vi "Initialize File Transfer Behavior.vi"(8 "error in (no error)":errorcluster, 11 "RT Management in":refnum<class "RT Management.lvclass">) -> (0 "error out":errorcluster, 2 "File Transfer Behavior out":refnum<class "File Transfer Behavior.lvclass">, 3 "RT Management out":refnum<class "RT Management.lvclass">)   [LabVIEW 2016, in "RT Management.lvlib" / "RT Management.lvclass"]
doc: "Initializes the appropriate File Transfer Behavior for the given target."
uses:
  RT Management.lvclass
  File Transfer Behavior/File Transfer Behavior.lvclass
  RT Management.lvclass/RT Management.ctl
  FTP/FTP.lvclass
  C:/GitHub/SystemManagementAndInformation/source/classes/File Transfer Behavior/File Transfer Behavior.lvclass
  WebDAV/WebDAV.lvclass
  Get File transfer behavior.vi
  Get Password.vi
  Get Username.vi
  Get Address.vi
  Set File Transfer Behavior.lvclass.vi
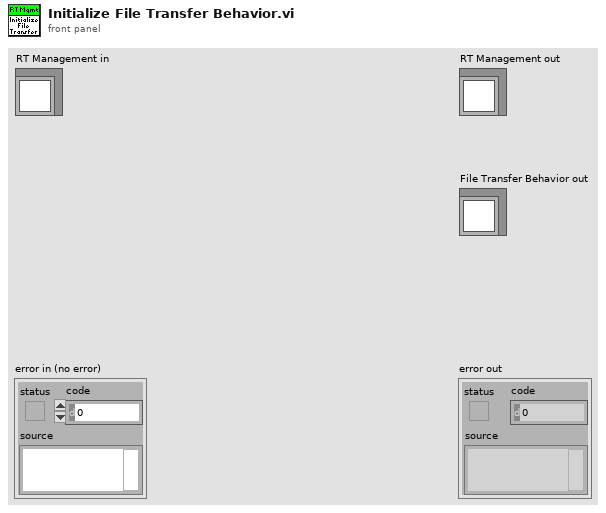
[diagram p1: front panel]
types:
  T1 = typedef "RT Management.lvlib/RT Management.lvclass/Operating system.ctl" = enum16{"Unknown", "VxWorks", "PharLap", "Linux-ARM", "Linux-x64"}
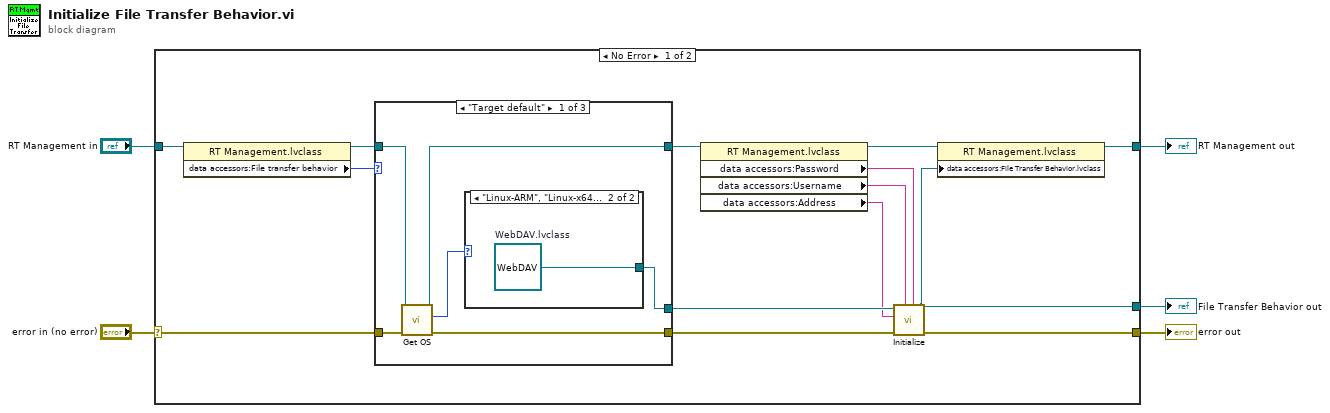
[diagram p0: block diagram]
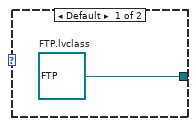
[diagram p2: hidden frame]
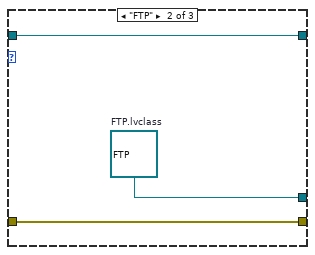
[diagram p3: hidden frame]
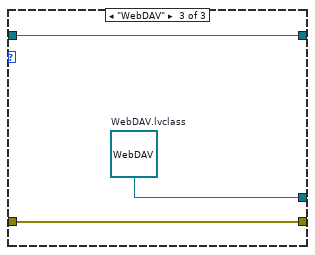
[diagram p4: hidden frame]
diagram:
  n1 = case shown="No Error" "error in (no error)" {
    selector: "error in (no error)" -> [w19 w35]
    tunnel: [w13 w35] -> w4
    tunnel: [w18 w34] -> w2
    tunnel: "RT Management in" -> [w17 w34]
    tunnel: [w6 _] -> w1
    frame No Error {
      n2 = property class="RT Management.lvclass"(reference=w17) -> (reference out=w15:refnum<class "RT Management.lvclass">, "data accessors:File transfer behavior"=w16:enum16{"Target default", "FTP", "WebDAV"})  [unwired: 1 in, 1 out]
      n3 = case shown="\"Target default\"" w16 {
        tunnel: w19 -> [w25 w28 w31]
        tunnel: [w21 w28 w31] -> w14
        tunnel: [w20 w29 w32] -> w12
        tunnel: w15 -> [w22 w30 w33]
        tunnel: [w23 w30 w33] -> w11
        frame "Target default" {
          n4 = call "Get OS.vi"("error in (no error)"=w25, "RT Management in"=w22) -> ("error out"=w21:errorcluster, "Operating System"=w24:T1, "RT Management out"=w23:refnum<class "RT Management.lvclass">)  [unwired: 6 in, 1 out]
          n5 = case shown="\"Linux-ARM\", \"Linux-x64\"" w24 {
            tunnel: [w26 w27] -> w20
            frame Default {
              w26 = refnum<class "FTP.lvclass"> refnum  # FTP.lvclass
            }
            frame "Linux-ARM", "Linux-x64" {
              w27 = refnum<class "WebDAV.lvclass"> refnum  # WebDAV.lvclass
            }
          }
        }
        frame "FTP" {
          w29 = refnum<class "FTP.lvclass"> refnum  # FTP.lvclass
        }
        frame "WebDAV" {
          w32 = refnum<class "WebDAV.lvclass"> refnum  # WebDAV.lvclass
        }
      }
      n6 = property class="RT Management.lvclass"(reference=w11) -> (reference out=w10:refnum<class "RT Management.lvclass">, "data accessors:Password"=w7:string, "data accessors:Username"=w8:string, "data accessors:Address"=w9:string)  [unwired: 1 in, 1 out]
      n7 = call-dynamic "Initialize.vi"("Password"=w7, "Username"=w8, "error in (no error)"=w14, "Address"=w9, "File Transfer Behavior in"=w12) -> ("error out"=w13:errorcluster, "File Transfer Behavior out"=w6:refnum<class "File Transfer Behavior.lvclass">)  [unwired: 5 in]
      n8 = property class="RT Management.lvclass"(reference=w10, "data accessors:File Transfer Behavior.lvclass"=w6) -> (reference out=w18:refnum<class "RT Management.lvclass">)  [unwired: 1 in, 1 out]
    }
    frame Error {
    }
  }
  "error out" <- w4
  "RT Management out" <- w2
  "File Transfer Behavior out" <- w1
